vi "File.Build FIle Name with Timestamp.vi"(10 "Sufix":string, 11 "File Name":string) -> (2 "Time Stamp Out":string, 3 "File Name Out":string)   [LabVIEW 2018]
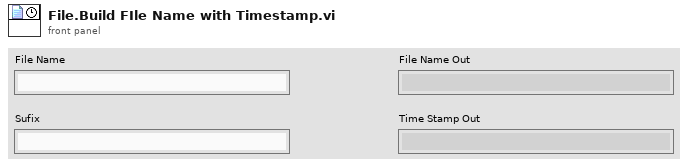
[diagram p1: front panel]
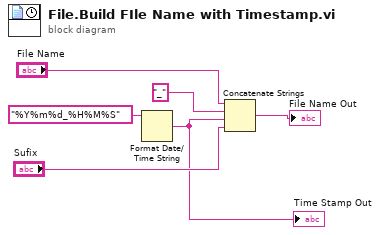
[diagram p0: block diagram]
diagram:
  n1 = Format Date/Time String(time format string (%c)="%Y%m%d_%H%M%S") -> (date/time string=w3:string)  [unwired: 2 in]
  "Time Stamp Out" <- w3
  n2 = Concatenate Strings("File Name", "_" ("time format string (%c)"), w3, "Sufix") -> (→"File Name Out":string)
